vi "Basic Averaged DC-RMS for N Chan.vi"(7 "reset":bool, 8 "error in (no error)":errorcluster, 9 "window":T1(ring), 10 "averaging type":enum16{"Linear", "Exponential"}(ring), 11 "signals in":waveform(dbl)[](array[waveform])) -> (0 "error out":errorcluster, 2 "RMS values":dbl[](array[numeric]) format="%.2p", 3 "DC values":dbl[](array[numeric]) format="%.2p", 4 "measurements info":T2(array[cluster]) {"uncertainty" format="%0.2p"})   [LabVIEW 2022 SP3, in "NI_MAPro.lvlib"]
doc: "Calculates the DC and RMS values of an input waveform or array of waveforms. This VI is similar to the Averaged DC-RMS VI, but this VI returns only one <B>DC value</B> and one <B>RMS value</B> per input waveform."
uses:
  NI_MAPro.lvlib
  NI_MABase.lvlib
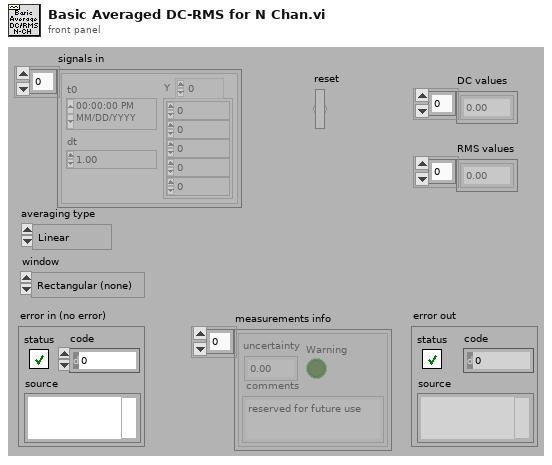
[diagram p1: front panel]
types:
  T1 = enum16{"Rectangular (none)", "Hanning", "Low side lobe"}
  T2 = cluster{"uncertainty":dbl, "Warning":bool, "comments":string}[]
  T3 = cluster{"DC history":dbl, "RMS history":dbl, "exp TC (samples)":dbl, "buffer size":i32, "t0 history":timestamp, "dt history":dbl, "timestamp":timestamp, "buffer":dbl[]}
  T4 = cluster{"uncertainty":dbl, "Warning":bool, "comments":string}
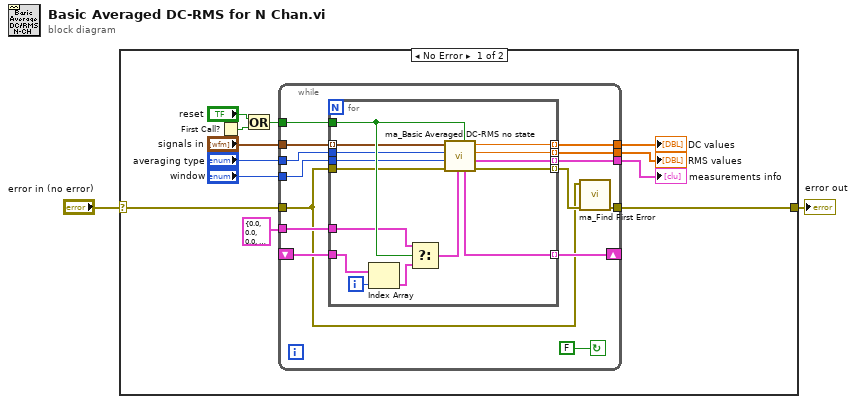
[diagram p0: block diagram]
diagram:
  n1 = case shown="No Error" "error in (no error)" {
    selector: "error in (no error)" -> [w4 w44]
    tunnel: [w5 w44] -> w1
    frame No Error {
      n2 = First Call?() -> (First Call?: T/F=w11:bool)
      n3 = Or(x="reset", y=w11) -> (x .or. y?=w9:bool)
      n4 = while {
        tunnel: [w21] -> w6
        tunnel: [w22] -> w7
        tunnel: [w23] -> w8
        tunnel: w9 -> [w28]
        shift-left: _ -> [w19]
        shift-right: [w24] -> _
        tunnel: "window" -> [w25]
        tunnel: "averaging type" -> [w26]
        tunnel: "signals in" -> [w27]
        tunnel: [w17] -> w5
        tunnel: w4 -> [w15]
        tunnel: T3 {"DC history"=0.0, "RMS history"=0.0, "exp TC (samples)"=0.0, "buffer size"=0, "t0 history"=timestamp(0 s since 1904-01-01), "dt history"=0.0, "timestamp"=timestamp(0 s since 1904-01-01), "buffer"=[]} ("state info") -> [w16]
        stop <- FALSE continue-if-true
        n5 = for {
          tunnel: w28 -> [w43]
          tunnel: w27 -> [w42] mode=indexing
          tunnel: w26 -> [w41]
          tunnel: w25 -> [w40]
          tunnel: [w39] -> w24 mode=indexing
          tunnel: [w38] -> w23 mode=indexing
          tunnel: [w37] -> w22 mode=indexing
          tunnel: [w36] -> w21 mode=indexing
          tunnel: w19 -> [w32]
          tunnel: [w34] -> w18 mode=indexing
          tunnel: w15 -> [w30]
          tunnel: w16 -> [w29]
          i -> [w33]
          n6 = Index Array(array=w32, index=w33) -> (element=w31:T3)
          n7 = Select(t=w29, s=w43, f=w31) -> (s? t:f=w35:T3)
          n8 = call "ma_Basic Averaged DC-RMS no state.vi"("reset"=w43, "state info"=w35, "error in"=w30, "window"=w40, "averaging type"=w41, "signal in"=w42) -> ("error out"=w34:errorcluster, "measurement info cluster"=w38:T4, "RMS value"=w36:dbl, "DC value"=w37:dbl, "state info"=w39:T3)  [unwired: 1 in]
        }
        n9 = call "ma_Find First Error.vi"("error array in"=w18, "error in 1 (no error)"=w15) -> ("error out"=w17:errorcluster)  [unwired: 5 in]
      }
      "DC values" <- w7
      "RMS values" <- w6
      "measurements info" <- w8
    }
    frame Error {
    }
  }
  "error out" <- w1
